vi "FPGA main.vi"() -> ()   [LabVIEW 2020]
uses:
  <vilib>/rvi/Emulation/niFpgaGetClockAttributes.vi
  <vilib>/rvi/Emulation/niFpgaSctlEmulationGetInTimedLoop.vi
  <vilib>/rvi/Emulation/niFpgaEmulationReportErrorSimple.vi
  <vilib>/rvi/eio/common/nirviEmuTemplateMethod_errors.vi
  <vilib>/rvi/eio/common/nirviEmuTemplatePropertySet_noerrors.vi
  <vilib>/rvi/eio/common/nirviEmuTemplatePropertyGet_noerrors.vi
  <vilib>/rvi/Emulation/niFpgaCriticalErrorInLSC.vi
  <vilib>/eio/EIONode/EIONode.xnode
  <vilib>/eio/EIOPropertyNode/EIOPropertyNode.xnode
  <vilib>/rvi/eio/common/nirviEmuTemplatePropertyGet_errors.vi
  <vilib>/rvi/eio/common/nirviEmuTemplatePropertySet_errors.vi
panel:
  out "Lock-in Amplitude":i16
  out "Lock-in Phase":i16
  out "AI4 Calibration Constants":cluster{u32, i32}={320529, -705996}
  out "AI0 Calibration Constants":cluster{u32, i32}={32044, -532}
  out "AI1 Calibration Constants":cluster{u32, i32}={32045, -62449}
  out "AI2 Calibration Constants":cluster{u32, i32}={320465, 78963}
  out "AI3 Calibration Constants":cluster{u32, i32}={320524, -422194}
  out "AO1 Calibration Constants":cluster{u32, i32}={310026, -619723}
  out "AO2 Calibration Constants":cluster{u32, i32}={310062, 882078}
  out "AO3 Calibration Constants":cluster{u32, i32}={310041, 2159970}
  in  "A0 Voltage Range":T1(ring)=enum."+/- 1 V"
  in  "A1 Voltage Range":T1(ring)=enum."+/- 1 V"
  in  "A2 Voltage Range":T1(ring)
  in  "A3 Voltage Range":T1(ring)
  in  "A4 Voltage Range":T1(ring)
  out "AO0 Calibration Constants":cluster{u32, i32}={310026, -619723}
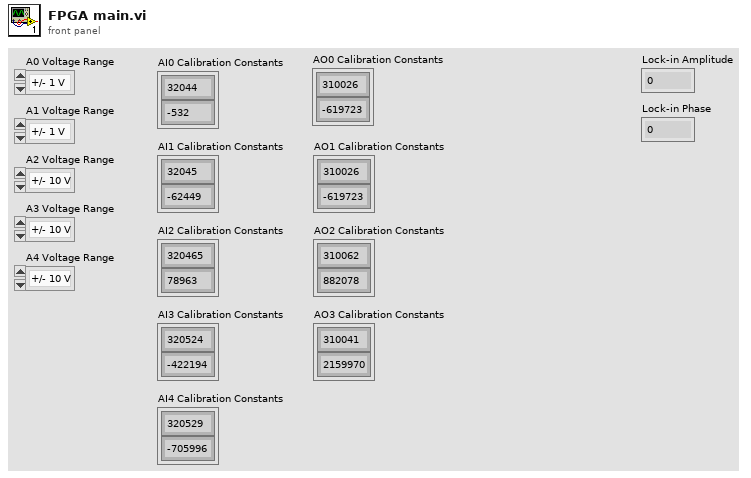
[diagram p1: front panel]
types:
  T1 = enum8{"+/- 10 V", "+/- 5 V", "+/- 2 V", "+/- 1 V"}
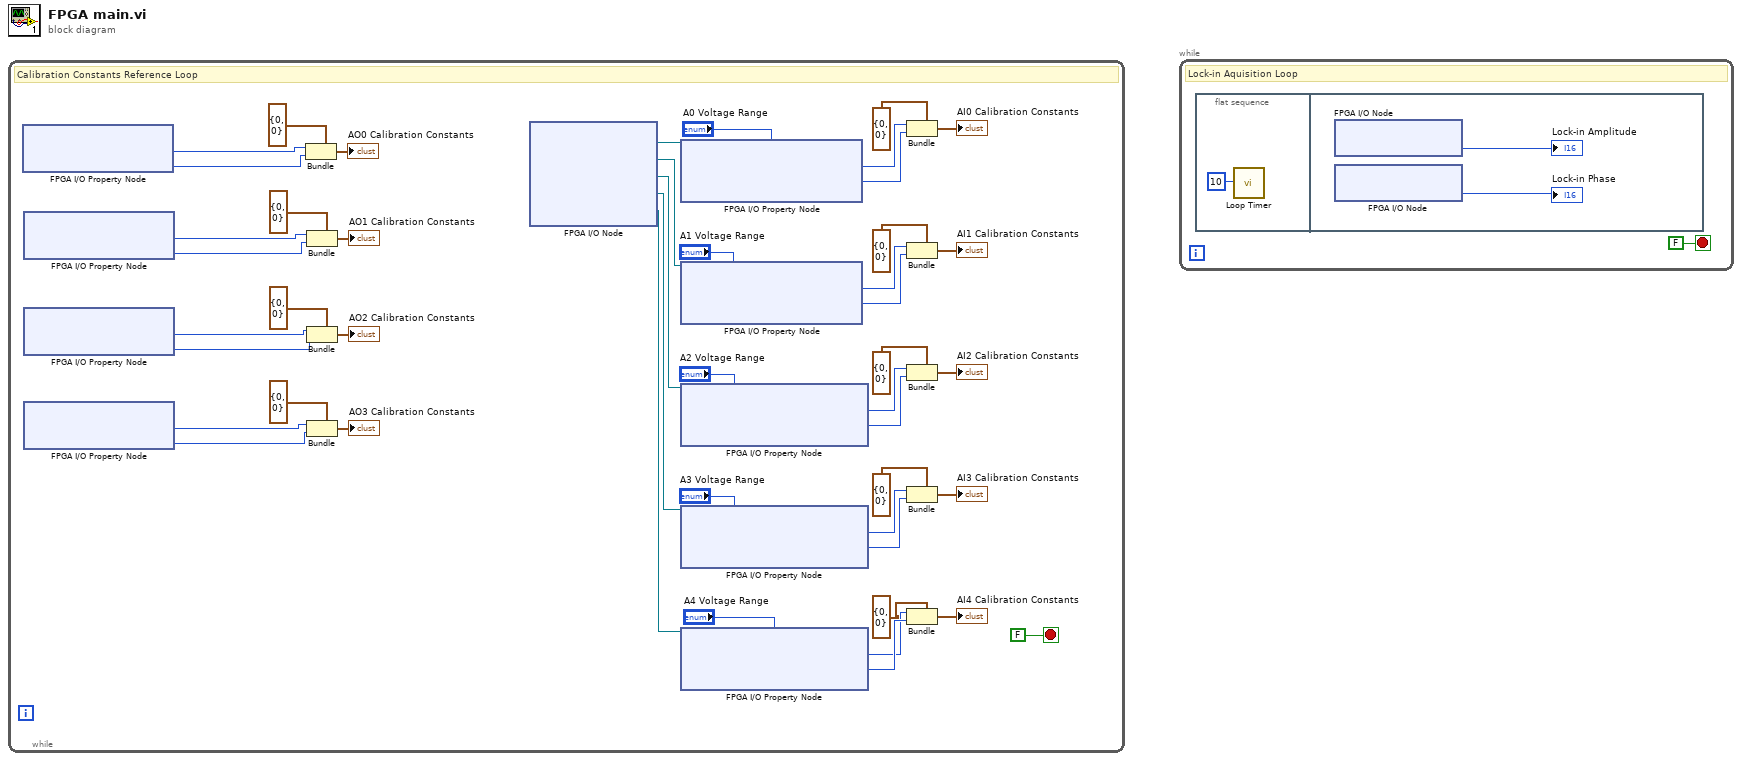
[diagram p0: block diagram]
diagram:
  n1 = while {
    stop <- FALSE stop-if-true
    # "Calibration Constants Reference Loop"
    n2 = xnode "FPGA I/O Property Node"() -> ("LSB Weight"=w2:u32, "Offset"=w3:i32)  [unwired: 1 in, 1 out]
    n3 = xnode "FPGA I/O Property Node"() -> ("LSB Weight"=w23:u32, "Offset"=w22:i32)  [unwired: 1 in, 1 out]
    n4 = xnode "FPGA I/O Property Node"() -> ("LSB Weight"=w18:u32, "Offset"=w19:i32)  [unwired: 1 in, 1 out]
    n5 = xnode "FPGA I/O Property Node"() -> ("LSB Weight"=w15:u32, "Offset"=w14:i32)  [unwired: 1 in, 1 out]
    n6 = Bundle(cluster=cluster{u32, i32} {0, 0}, w2, w3) -> (→"AO0 Calibration Constants":cluster{u32, i32})
    n7 = Bundle(cluster=cluster{u32, i32} {0, 0}, w23, w22) -> (→"AO1 Calibration Constants":cluster{u32, i32})
    n8 = Bundle(cluster=cluster{u32, i32} {0, 0}, w18, w19) -> (→"AO2 Calibration Constants":cluster{u32, i32})
    n9 = Bundle(cluster=cluster{u32, i32} {0, 0}, w15, w14) -> (→"AO3 Calibration Constants":cluster{u32, i32})
    n10 = xnode "FPGA I/O Node"() -> ("FPGA I/O Out"=w40:refnum<k21>, "FPGA I/O Out"=w28:refnum<k21>, "FPGA I/O Out"=w27:refnum<k21>, "FPGA I/O Out"=w26:refnum<k21>, "FPGA I/O Out"=w25:refnum<k21>)  [unwired: 5 in, 5 out]
    n11 = xnode "FPGA I/O Property Node"("FPGA I/O In"=w40, "Voltage Range"="A0 Voltage Range") -> ("LSB Weight (+/- 1 V range)"=w42:u32, "Offset (+/- 1 V range)"=w43:i32)  [unwired: 1 out]
    n12 = xnode "FPGA I/O Property Node"("FPGA I/O In"=w28, "Voltage Range"="A1 Voltage Range") -> ("LSB Weight (+/- 1 V range)"=w45:u32, "Offset (+/- 1 V range)"=w44:i32)  [unwired: 1 out]
    n13 = xnode "FPGA I/O Property Node"("FPGA I/O In"=w27, "Voltage Range"="A2 Voltage Range") -> ("LSB Weight (+/- 10 V range)"=w34:u32, "Offset (+/- 10 V range)"=w35:i32)  [unwired: 1 out]
    n14 = xnode "FPGA I/O Property Node"("FPGA I/O In"=w26, "Voltage Range"="A3 Voltage Range") -> ("LSB Weight (+/- 10 V range)"=w30:u32, "Offset (+/- 10 V range)"=w29:i32)  [unwired: 1 out]
    n15 = xnode "FPGA I/O Property Node"("FPGA I/O In"=w25, "Voltage Range"="A4 Voltage Range") -> ("LSB Weight (+/- 10 V range)"=w37:u32, "Offset (+/- 10 V range)"=w38:i32)  [unwired: 1 out]
    n16 = Bundle(cluster=cluster{u32, i32} {0, 0}, w42, w43) -> (→"AI0 Calibration Constants":cluster{u32, i32})
    n17 = Bundle(cluster=cluster{u32, i32} {0, 0}, w45, w44) -> (→"AI1 Calibration Constants":cluster{u32, i32})
    n18 = Bundle(cluster=cluster{u32, i32} {0, 0}, w34, w35) -> (→"AI2 Calibration Constants":cluster{u32, i32})
    n19 = Bundle(cluster=cluster{u32, i32} {0, 0}, w30, w29) -> (→"AI3 Calibration Constants":cluster{u32, i32})
    n20 = Bundle(cluster=cluster{u32, i32} {0, 0}, w37, w38) -> (→"AI4 Calibration Constants":cluster{u32, i32})
  }
  n21 = while {
    stop <- FALSE stop-if-true
    # "Lock-in Aquisition Loop"
    n22 = flat-sequence {
      frame #0 {
        n23 = call "Loop Timer"("Count(uSec)"=u16 10) -> ()  [unwired: 1 out]
      }
      frame #1 {
        n24 = xnode "FPGA I/O Node"() -> ("Connector1/AI2"=→"Lock-in Amplitude":i16)  [unwired: 1 in, 1 out]
        n25 = xnode "FPGA I/O Node"() -> ("Connector1/AI3"=→"Lock-in Phase":i16)  [unwired: 1 in, 1 out]
      }
    }
  }
